vi "Distance-Velocity from Freq.vi"(0 "freq_rising":dbl, 2 "Empirical Distance Costant":dbl=4.28571429e-07 format="%#_13g", 3 "freq_falling":dbl) -> (5 "Distance (m)":dbl, 6 "Mean Frequency":dbl, 7 "Velocity (m/s)":dbl)   [LabVIEW 2014]
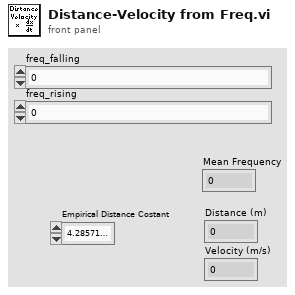
[diagram p1: front panel]
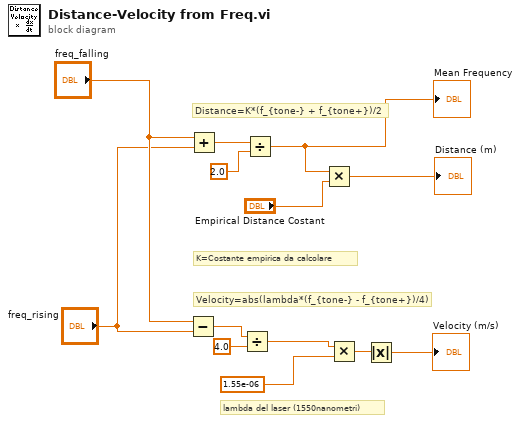
[diagram p0: block diagram]
diagram:
  # "Velocity=abs(lambda*(f_{tone-} - f_{tone+})/4)"
  # "Distance=K*(f_{tone-} + f_{tone+})/2"
  # "lambda del laser (1550nanometri)"
  # "K=Costante empirica da calcolare"
  n1 = Subtract(x="freq_falling", y="freq_rising") -> (x-y=w8:dbl)
  n2 = Add(x="freq_falling", y="freq_rising") -> (x+y=w13:dbl)
  n3 = Divide(x=w8, y=4.0) -> (x/y=w6:dbl)
  n4 = Divide(x=w13, y=2.0) -> (x/y=w11:dbl)
  "Mean Frequency" <- w11
  n5 = Multiply(x=w11, y="Empirical Distance Costant") -> (x*y=→"Distance (m)":dbl)
  n6 = Multiply(x=w6, y=1.55e-06) -> (x*y=w2:dbl)
  n7 = Absolute Value(x=w2) -> (abs(x)=→"Velocity (m/s)":dbl)
